vi "Send VISA Param.vi"(8 "error in (no error)":errorcluster, 11 "Server in":refnum<class "Server.lvclass">) -> (0 "error out":errorcluster, 3 "Server out":refnum<class "Server.lvclass">)   [LabVIEW 2018, in "Server.lvclass"]
uses:
  Server.lvclass
  Server.lvclass/Server.ctl
panel:
  out "Output Cluster":T1={"baud rate (9600)"=2400, "VISA resource name"=""}
  in  "Input Cluster":T1={"baud rate (9600)"=2400, "VISA resource name"=""}
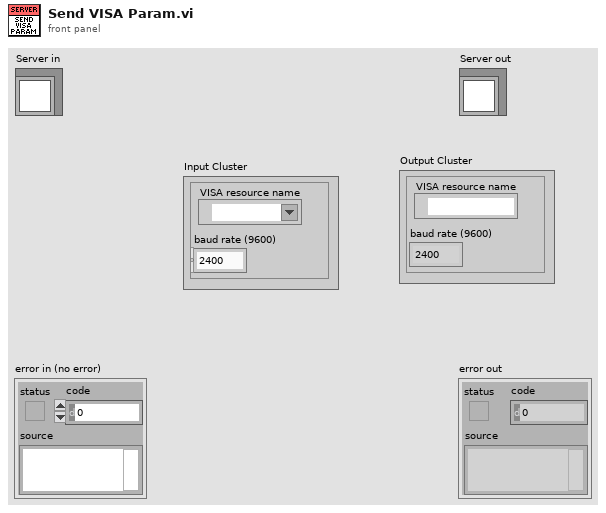
[diagram p1: front panel]
types:
  T1 = cluster{"baud rate (9600)":u32, "VISA resource name":refnum<visa-resource-name>}
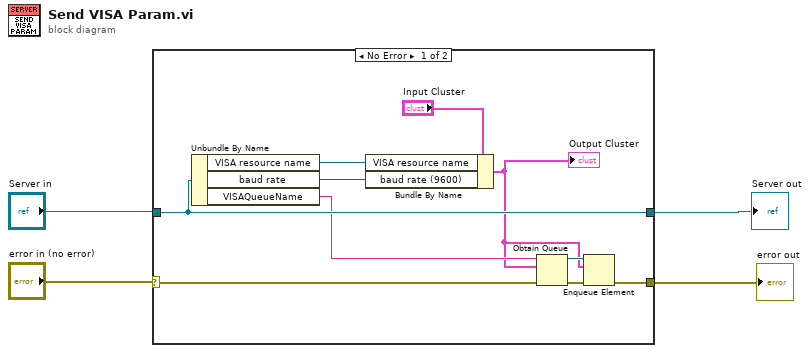
[diagram p0: block diagram]
diagram:
  n1 = case shown="No Error" "error in (no error)" {
    selector: "error in (no error)" -> [w10 w16]
    tunnel: [w12 w16] -> w1
    tunnel: [w11 w15] -> w2
    tunnel: "Server in" -> [w11 w15]
    frame No Error {
      n2 = Unbundle By Name(w11) -> ("VISA resource name"=w5:refnum<visa-resource-name>, "baud rate"=w7:u32, "VISAQueueName"=w9:string)
      n3 = Bundle By Name(cluster="Input Cluster", "VISA resource name"=w5, "baud rate (9600)"=w7) -> (w6:T1)
      "Output Cluster" <- w6
      n4 = Obtain Queue(name (unnamed)=w9, element data type=w6, error in (no error)=w10) -> (queue out=w14:refnum<queue>, error out=w13:errorcluster)  [unwired: 2 in, 1 out]
      n5 = Enqueue Element(queue=w14, element=w6, error in (no error)=w13) -> (error out=w12:errorcluster)  [unwired: 1 in, 2 out]
    }
    frame Error {
    }
  }
  "error out" <- w1
  "Server out" <- w2
